vi "XY Graph Rotate Plot.vi"(6 "t_0 (NaN: use index)":dbl=nan, 8 "Error In":errorcluster, 9 "Index of t_0":i32, 11 "Decay in":cluster{"t Array":dbl[], "I Array":dbl[]}) -> (0 "Error Out":errorcluster, 1 "t_0":dbl, 3 "Decay out":cluster{"t Array":dbl[], "I Array":dbl[]})   [LabVIEW 2021, in "XY Graph Add-Ons.lvlib"]
uses:
  XY Graph Add-Ons.lvlib
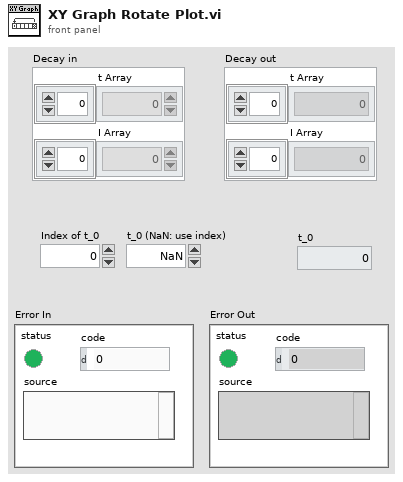
[diagram p1: front panel]
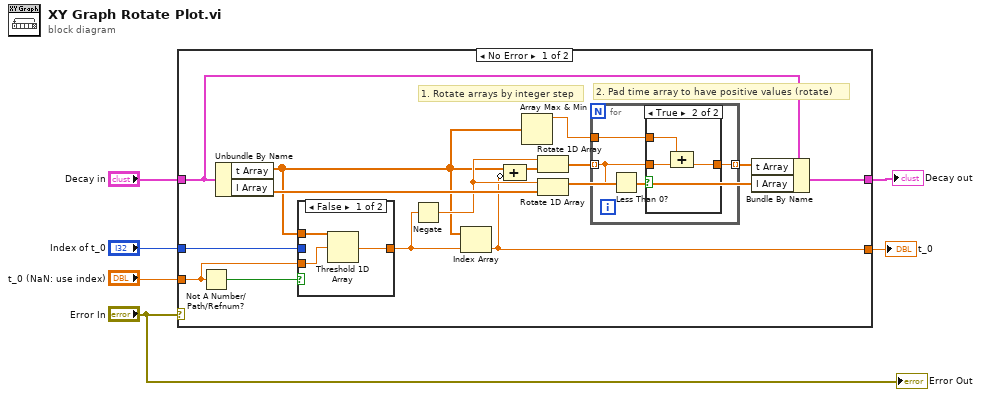
[diagram p0: block diagram]
diagram:
  n1 = case shown="No Error" "Error In" {
    tunnel: "Decay in" -> [w20 w35]
    tunnel: [w15 w34] -> w5
    tunnel: [w13 w35] -> w4
    tunnel: "Index of t_0" -> [w10 _]
    tunnel: "t_0 (NaN: use index)" -> [w7 w34]
    frame No Error {
      # "2. Pad time array to have positive values (rotate)"
      # "1. Rotate arrays by integer step"
      n2 = Not A Number/Path/Refnum?(number/path/refnum=w7) -> (NaN/Path/Refnum?=w11:bool)
      n3 = Unbundle By Name(w20) -> ("t Array"=w8:dbl[], "I Array"=w21:dbl[])
      n4 = case shown="False" w11 {
        tunnel: [w22 w25] -> w9
        tunnel: w10 -> [_ w25]
        tunnel: w8 -> [w24 _]
        tunnel: w7 -> [w23 _]
        frame False {
          n5 = Threshold 1D Array(2:w23, 3:w24) -> (0:w22:dbl)  [unwired: 1 in]
        }
        frame True {
        }
      }
      n6 = Negate(x=w9) -> (-x=w19:dbl)
      n7 = Index Array(array=w8, index=w9) -> (element=w15:dbl)
      n8 = Compound Arithmetic op=ADD(w8, invert w15) -> (w14:dbl[])
      n9 = Array Max & Min(array=w8) -> (max value=w18:dbl)  [unwired: 3 out]
      n10 = Rotate 1D Array(1:w14, 2:w19) -> (0:w16:dbl[])
      n11 = Rotate 1D Array(1:w21, 2:w19) -> (0:w12:dbl[])
      n12 = for {
        tunnel: w16 -> [w28] mode=indexing
        tunnel: [w27] -> w17 mode=indexing
        tunnel: w18 -> [w26]
        n13 = Less Than 0?(x=w28) -> (x < 0?=w29:bool)
        n14 = case shown="True" w29 {
          tunnel: w28 -> [w30 w33]
          tunnel: [w30 w31] -> w27
          tunnel: w26 -> [_ w32]
          frame False {
          }
          frame True {
            n15 = Compound Arithmetic op=ADD(w32, w33) -> (w31:dbl)
          }
        }
      }
      n16 = Bundle By Name(cluster=w20, "t Array"=w17, "I Array"=w12) -> (w13:cluster{"t Array":dbl[], "I Array":dbl[]})
    }
    frame Error {
    }
  }
  "t_0" <- w5
  "Decay out" <- w4
  "Error Out" <- "Error In"
